vi "set_frame_rate.vi"(8 "error in (no error)":errorcluster, 10 "frame rate":dbl[unit]=1.0, 11 "MG090623BinningImageAssembler.lvclass in":refnum<class "ImageAssemblerMG090623Binning.lvclass">) -> (0 "error out":errorcluster, 3 "MG090623BinningImageAssembler.lvclass out":refnum<class "ImageAssemblerMG090623Binning.lvclass">)   [LabVIEW 2010, in "ImageAssemblerMG090623Binning.lvclass"]
uses:
  ImageAssemblerMG090623Binning.lvclass
  ImageAssemblerMG090623Binning.lvclass/ImageAssemblerMG090623Binning.ctl
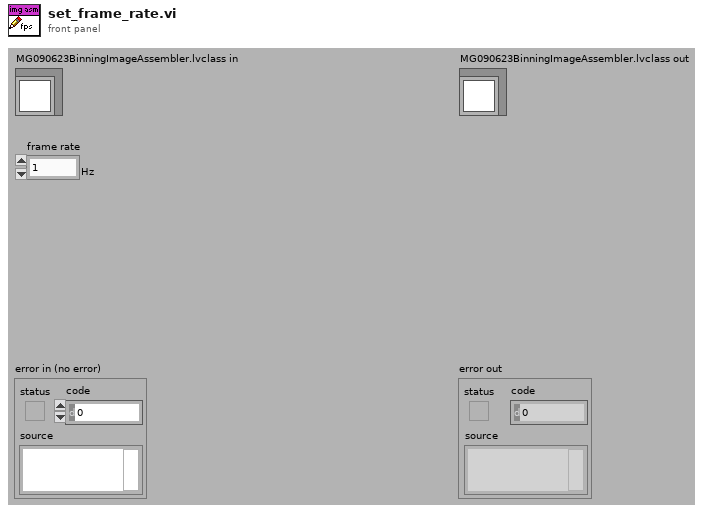
[diagram p1: front panel]
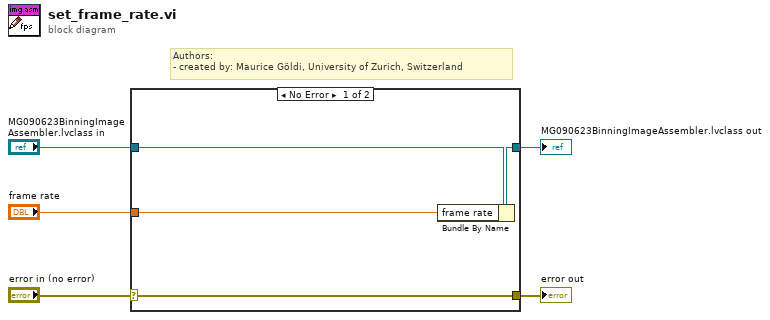
[diagram p0: block diagram]
diagram:
  # "Authors: \n- created by: Maurice Göldi, University of Zurich, Switzerland"
  n1 = case shown="No Error" "error in (no error)" {
    selector: "error in (no error)" -> [w9 w10]
    tunnel: [w9 w10] -> w4
    tunnel: [w7 w11] -> w2
    tunnel: "MG090623BinningImageAssembler.lvclass in" -> [w8 w11]
    tunnel: "frame rate" -> [w6 _]
    frame No Error {
      n2 = Bundle By Name(cluster=w8, "frame rate"=w6) -> (w7:refnum<class "ImageAssemblerMG090623Binning.lvclass">)
    }
    frame Error {
    }
  }
  "error out" <- w4
  "MG090623BinningImageAssembler.lvclass out" <- w2
